vi "WriterEStopFGV.vi"(7 "E-Stop Action":T1, 8 "Error In":errorcluster, 11 "E-Stop In":bool) -> (0 "Error Out":errorcluster, 3 "E-Stop Out":bool)   [LabVIEW 2011]
uses:
  EStopAction.ctl
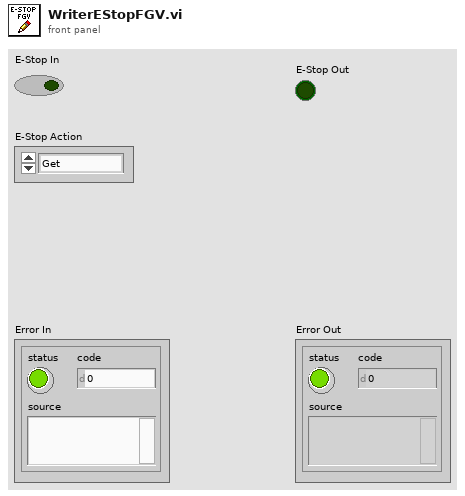
[diagram p1: front panel]
types:
  T1 = typedef "EStopAction.ctl" = enum16{"Get", "Set"}
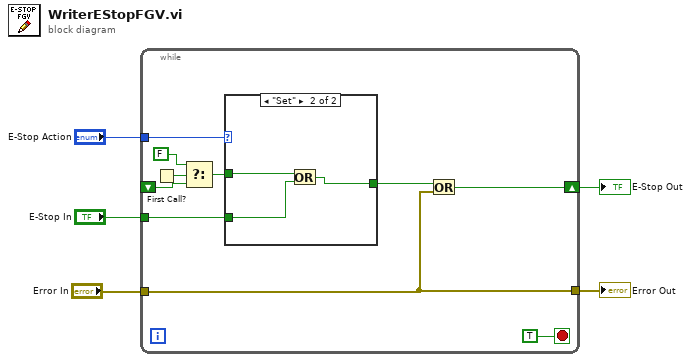
[diagram p0: block diagram]
diagram:
  n1 = while {
    tunnel: "E-Stop Action" -> [w14]
    tunnel: "E-Stop In" -> [w13]
    shift-right: [w7] -> w2
    shift-left: _ -> [w11]
    tunnel: "Error In" -> [w6]
    tunnel: [w6] -> w1
    stop <- TRUE stop-if-true
    n2 = First Call?() -> (First Call?: T/F=w12:bool)
    n3 = Select(t=FALSE, s=w12, f=w11) -> (s? t:f=w9:bool)
    n4 = case shown="\"Set\"" w14 {
      tunnel: w13 -> [_ w19]
      tunnel: w9 -> [w16 w18]
      tunnel: [w16 w17] -> w8
      frame "Get", Default {
      }
      frame "Set" {
        n5 = Or(x=w18, y=w19) -> (x .or. y?=w17:bool)
      }
    }
    n6 = Or(x=w8, y=w6) -> (x .or. y?=w7:bool)
  }
  "Error Out" <- w1
  "E-Stop Out" <- w2
